vi "Read Config Cameras.vi"(8 "error in":errorcluster, 11 "Config Manager in":refnum<class "Config Manager Class.lvclass">) -> (0 "error out":errorcluster, 1 "Camera Enums":T1[](array[typedef]), 2 "IMAQdx Cameras":T2(array[cluster]), 3 "Config Manager out":refnum<class "Config Manager Class.lvclass">)   [LabVIEW 2017, in "Config Manager Class.lvclass"]
uses:
  Config Manager Class.lvclass
  Type Definitions/Camera Enum.ctl
  Config Manager Class.lvclass/Config Manager Class.ctl
  <vilib>/Utility/config.llb/Read Key (String).vi
  <vilib>/Utility/config.llb/NI_LVConfig.lvlib
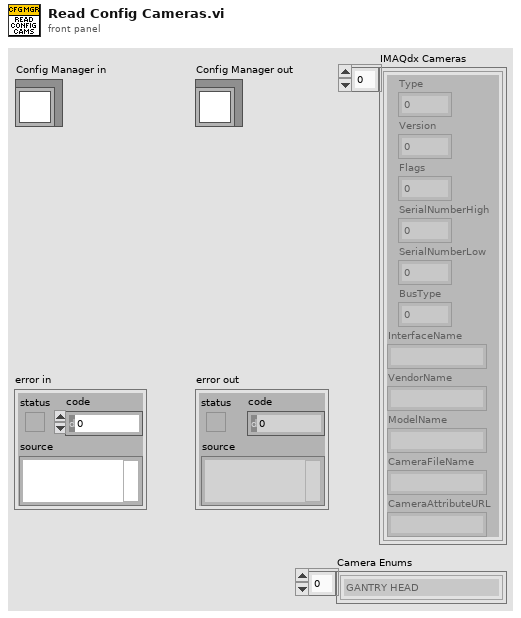
[diagram p1: front panel]
types:
  T1 = typedef "Camera Enum.ctl" = enum16{"GANTRY HEAD", "NEEDLE CALIBRATION X", "NEEDLE CALIBRATION Y", "STAND CAMERA", "SIMRAN WEBCAM"}
  T2 = cluster{"Type":u32, "Version":u32, "Flags":u32, "SerialNumberHigh":u32, "SerialNumberLow":u32, "BusType":u32, "InterfaceName":string, "VendorName":string, "ModelName":string, "CameraFileName":string, "CameraAttributeURL":string}[]
  T3 = cluster{"Type":u32, "Version":u32, "Flags":u32, "SerialNumberHigh":u32, "SerialNumberLow":u32, "BusType":u32, "InterfaceName":string, "VendorName":string, "ModelName":string, "CameraFileName":string, "CameraAttributeURL":string}
  T4 = typedef "NI_LVConfig.lvlib/Config Data RefNum.ctl" = refnum<k1>
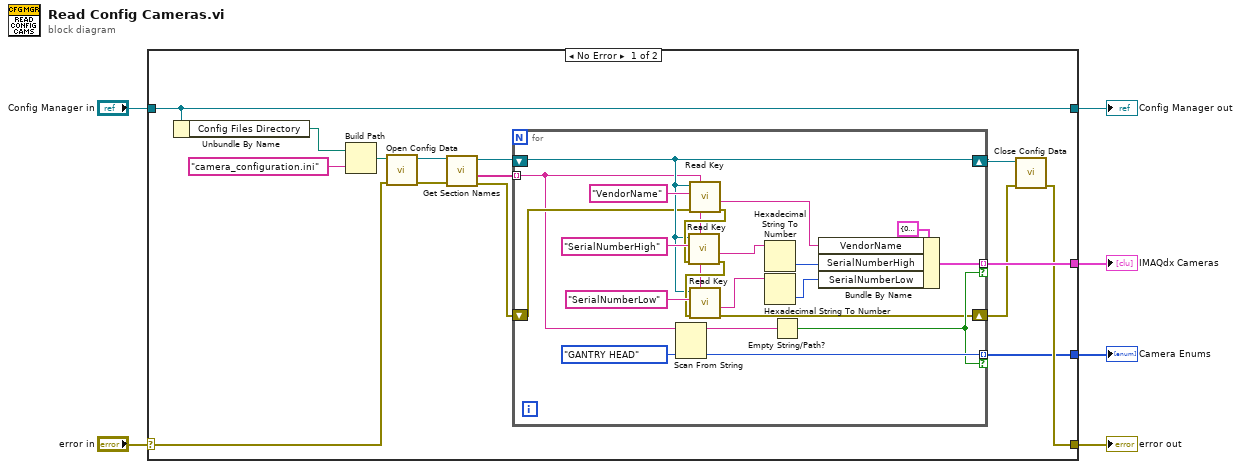
[diagram p0: block diagram]
diagram:
  n1 = case shown="No Error" "error in" {
    selector: "error in" -> [w14 w43]
    tunnel: [w8 w43] -> w5
    tunnel: [w16 w42] -> w3
    tunnel: "Config Manager in" -> [w16 w42]
    tunnel: [w11 _] -> w2
    tunnel: [w7 _] -> w1
    frame No Error {
      n2 = Unbundle By Name(w16) -> ("Config Files Directory"=w17:path)
      n3 = Build Path(base path=w17, name or relative path="camera_configuration.ini") -> (appended path=w20:path)
      n4 = call <vilib>:"Open Config Data.vi"("error in (no error)"=w14, "configuration file path"=w20) -> ("error out"=w19:errorcluster, "refnum"=w18:T4)  [unwired: 7 in, 1 out]
      n5 = call <vilib>:"Get Section Names.vi"("error in (no error)"=w19, "refnum"=w18) -> ("error out"=w10:errorcluster, "section names"=w15:string[], "refnum out"=w13:T4)  [unwired: 7 in]
      n6 = for {
        tunnel: w15 -> [w27] mode=indexing
        tunnel: [w25] -> w11 mode=indexing if=w23
        shift-right: [w22] -> w9
        shift-left: w10 -> [w29]
        tunnel: [w24] -> w7 mode=indexing if=w23
        shift-right: [w35] -> w12
        shift-left: w13 -> [w35]
        n7 = Scan From String(input string=w27, default 1=Camera_Enum."GANTRY HEAD" ("Camera")) -> (remaining string=w26:string, output 1=w24:T1)  [unwired: 3 in, 2 out]
        n8 = call-poly <vilib>:"Read Key.vi"("section"=w27, "error in (no error)"=w29, "key"="VendorName", "refnum"=w35) -> ("error out"=w38:errorcluster, "value"=w34:string)  [unwired: 4 in, 2 out]
        n9 = call-poly <vilib>:"Read Key.vi"("section"=w27, "error in (no error)"=w38, "key"="SerialNumberHigh", "refnum"=w35) -> ("error out"=w37:errorcluster, "value"=w33:string)  [unwired: 4 in, 2 out]
        n10 = call-poly <vilib>:"Read Key.vi"("section"=w27, "error in (no error)"=w37, "key"="SerialNumberLow", "refnum"=w35) -> ("error out"=w22:errorcluster, "value"=w32:string)  [unwired: 4 in, 2 out]
        n11 = Hexadecimal String To Number(string=w33) -> (number=w30:u32)  [unwired: 2 in, 1 out]
        n12 = Hexadecimal String To Number(string=w32) -> (number=w31:u32)  [unwired: 2 in, 1 out]
        n13 = Empty String/Path?(string/path=w26) -> (empty?=w23:bool)
        n14 = Bundle By Name(cluster=T3 {"Type"=0, "Version"=0, "Flags"=0, "SerialNumberHigh"=0, "SerialNumberLow"=0, "BusType"=0, "InterfaceName"="", "VendorName"="", "ModelName"="", "CameraFileName"="", "CameraAttributeURL"=""} ("IMAQdx Data"), "VendorName"=w34, "SerialNumberHigh"=w30, "SerialNumberLow"=w31) -> (w25:T3)
      }
      n15 = call <vilib>:"Close Config Data.vi"("error in (no error)"=w9, "refnum"=w12) -> ("error out"=w8:errorcluster)  [unwired: 8 in, 1 out]
    }
    frame Error {
    }
  }
  "error out" <- w5
  "Config Manager out" <- w3
  "IMAQdx Cameras" <- w2
  "Camera Enums" <- w1
